vi "main_feedback_sliders.vi"(9 "Running?":refnum<vi>, 10 "Inflow fractions":refnum<vi>, 11 "PH":refnum<vi>) -> ()   [LabVIEW 2019]
uses:
  lib/libSimulationControl/libSimulationControl.lvlib
  lib/libFileFunctions/libFileFunctions.lvlib
panel:
  out "ph_arr out":dbl[](array[numeric])
  out "reactorState files":string
  out "Fractions":dbl[](array[numeric])
  out "Values":i32[](array[numeric])
  out "Sum":i32
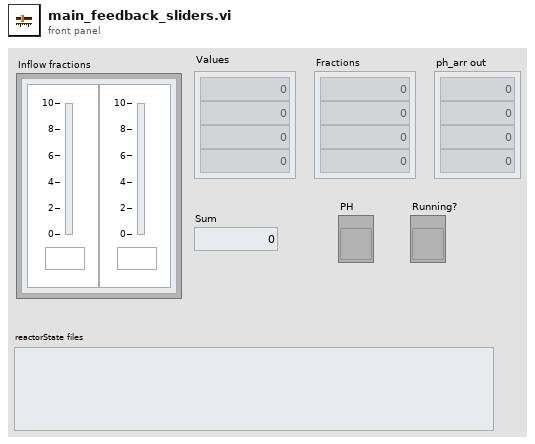
[diagram p1: front panel]
types:
  T1 = enum8{"Enabled", "Disabled", "Disabled and Grayed Out"}
  T2 = cluster{"Vertical Pointer Slide":i32, "String":string}
  T3 = cluster{"Vertical Pointer Slide":i32, "String":string}[]
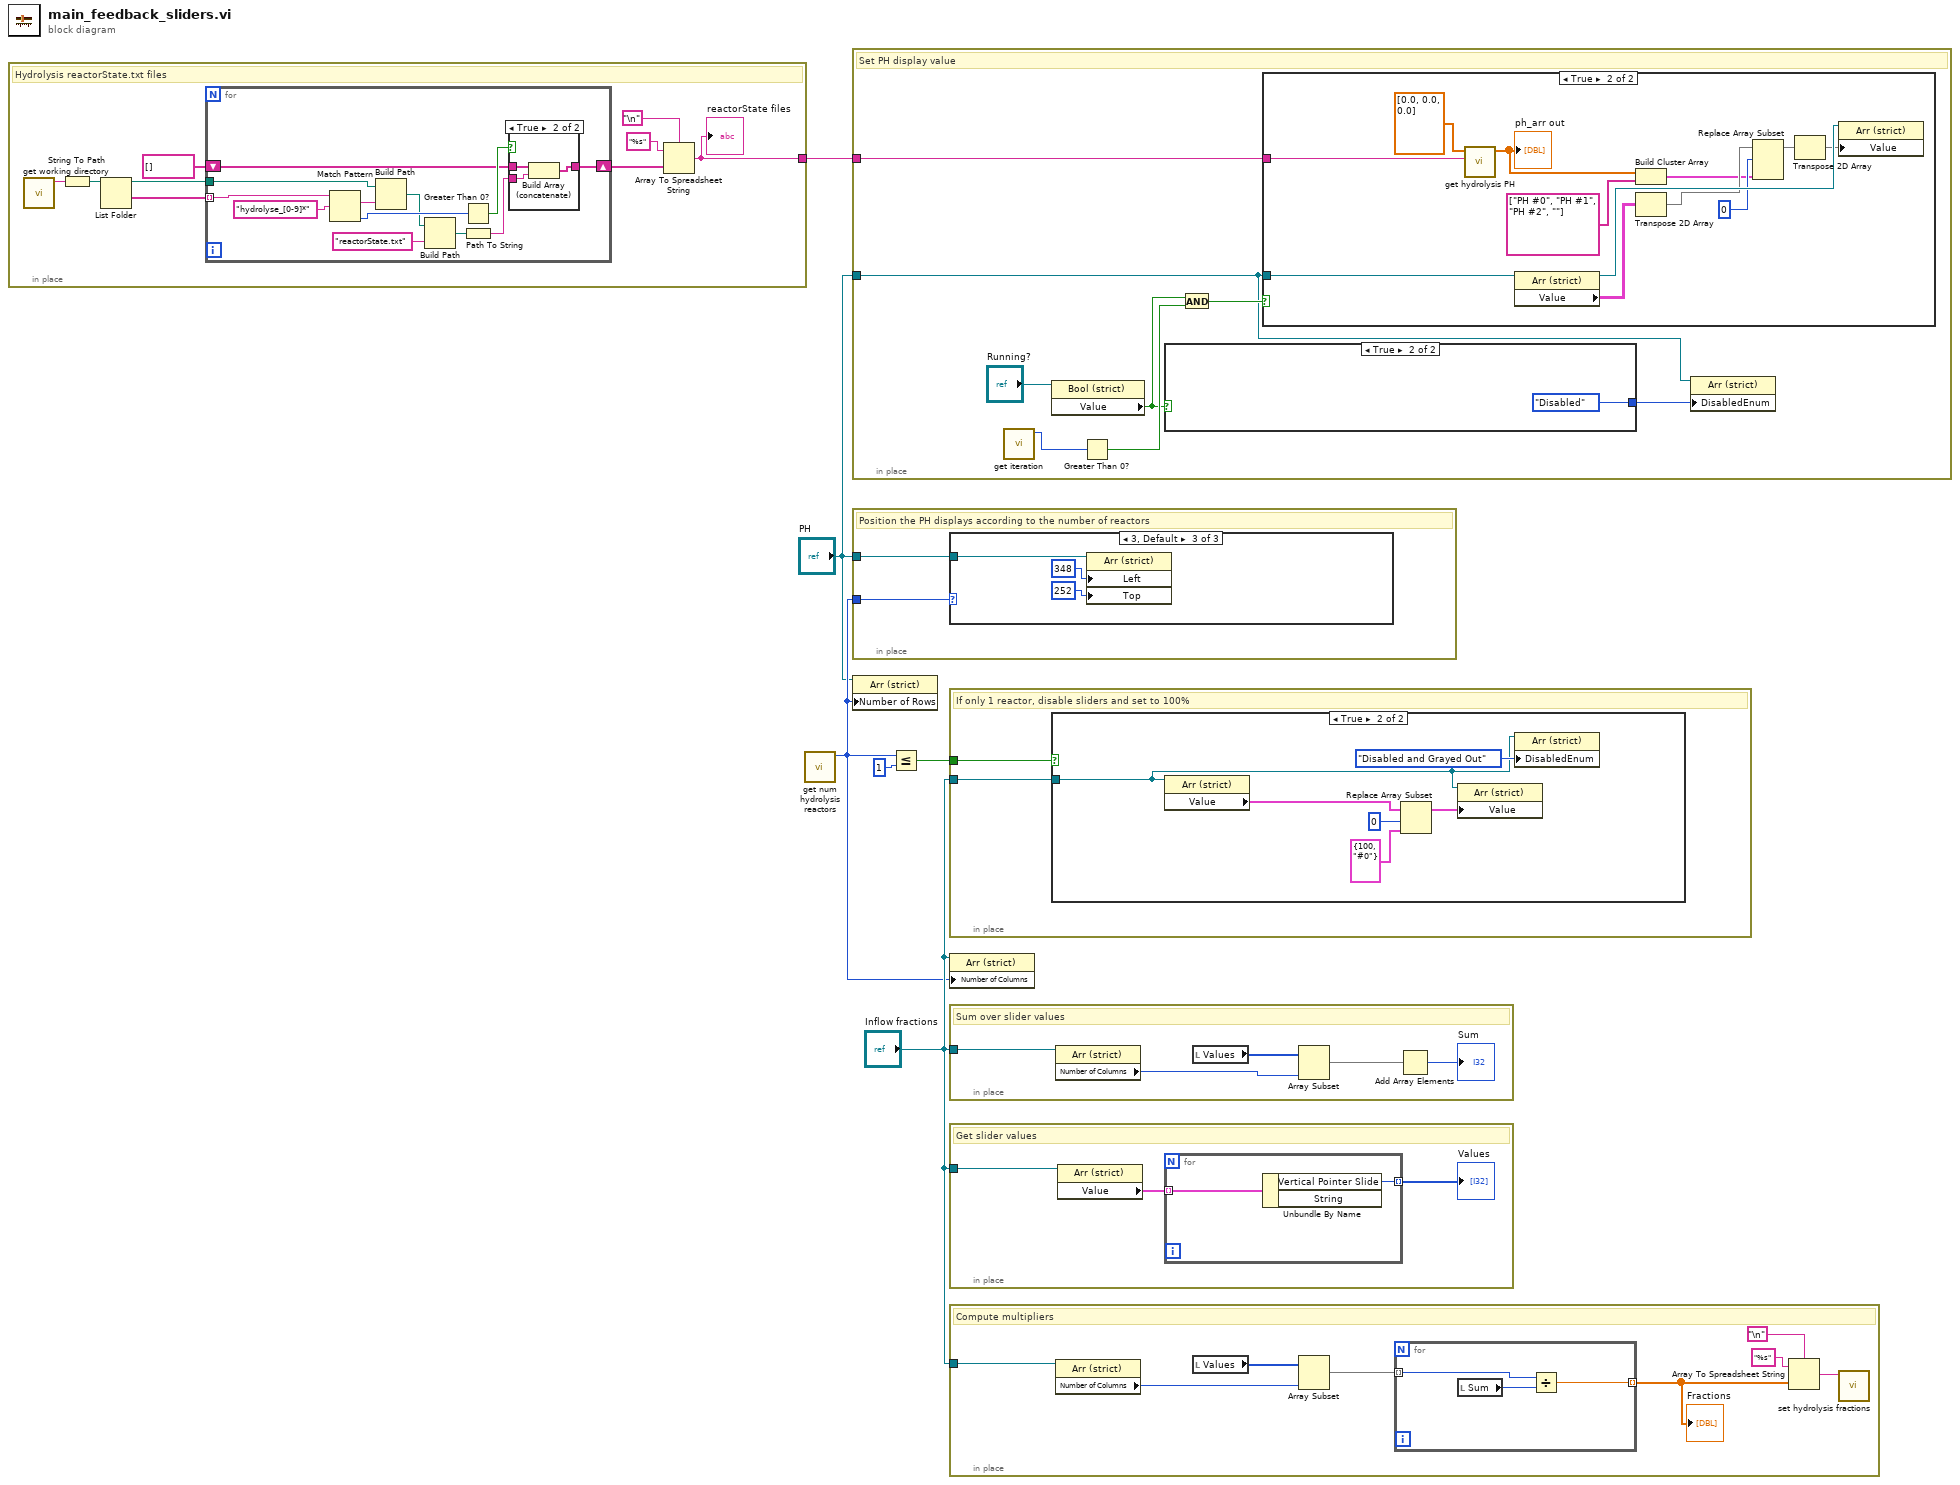
[diagram p0: block diagram]
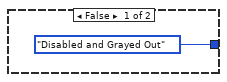
[diagram p3: hidden frame]
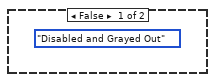
[diagram p4: hidden frame]
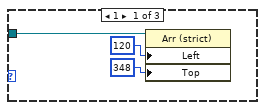
[diagram p5: hidden frame]
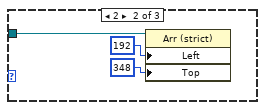
[diagram p6: hidden frame]
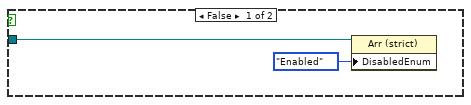
[diagram p7: hidden frame]
diagram:
  n1 = in-place {
    in-place-border: [w7] -> w1
    # "Hydrolysis reactorState.txt files"
    n2 = call "get working directory.vi"() -> ("function return"=w13:string)  [unwired: 10 in, 1 out]
    n3 = String To Path(string=w13) -> (path=w12:path)
    n4 = List Folder(path=w12) -> (path out=w11:path, folder names=w15:string[])  [unwired: 3 in, 2 out]
    n5 = for {
      tunnel: w15 -> [w22] mode=indexing
      shift-right: [w23] -> w10
      shift-left: string[] [] -> [w24]
      tunnel: w11 -> [w21]
      n6 = Match Pattern(string=w22, regular expression="hydrolyse_[0-9]*") -> (match substring=w20:string, offset past match=w25:i32)  [unwired: 1 in, 2 out]
      n7 = Build Path(base path=w21, name or relative path=w20) -> (appended path=w19:path)
      n8 = Build Path(base path=w19, name or relative path="reactorState.txt") -> (appended path=w17:path)
      n9 = Greater Than 0?(x=w25) -> (x > 0?=w26:bool)
      n10 = Path To String(path=w17) -> (string=w16:string)
      n11 = case shown="True" w26 {
        tunnel: [w28 w31] -> w23
        tunnel: w24 -> [w28 w30]
        tunnel: w16 -> [_ w29]
        frame False {
        }
        frame True {
          n12 = Build Array (concatenate)(w30, w29) -> (w31:string[])
        }
      }
    }
    n13 = Array To Spreadsheet String(delimiter (Tab)="\n", array=w10, 3:"%s" ("format string")) -> (spreadsheet string=w7:string)
    "reactorState files" <- w7
  }
  n14 = call "get num hydrolysis reactors.vi"() -> ("function return"=w3:i32)  [unwired: 10 in, 1 out]
  n15 = in-place {
    in-place-border: "PH" -> [w32]
    in-place-border: w1 -> [w36]
    # "Set PH display value"
    n16 = call "get iteration.vi"() -> ("function return"=w39:i32)  [unwired: 10 in, 1 out]
    n17 = property on="Property Node" class="Bool (strict)"(reference="Running?") -> ("Value"=w35:bool)  [unwired: 1 in, 2 out]
    n18 = Greater Than 0?(x=w39) -> (x > 0?=w38:bool)
    n19 = case shown="True" w35 {
      tunnel: [T1."Disabled and Grayed Out" ("Disabled") T1."Disabled" ("Disabled")] -> w34
      frame False {
      }
      frame True {
      }
    }
    n20 = And(x=w35, y=w38) -> (x .and. y?=w37:bool)
    n21 = case shown="True" w37 {
      tunnel: w32 -> [_ w53]
      tunnel: w36 -> [_ w43]
      frame False {
        (unwired) T1."Disabled and Grayed Out" ("Disabled")
      }
      frame True {
        n22 = call "get hydrolysis PH.vi"("reactor_state_files"=w43, "ph_arr 2"=dbl[] [0.0, 0.0, 0.0]) -> ("ph_arr out"=w44:dbl[])  [unwired: 8 in, 1 out]
        "ph_arr out" <- w44
        n23 = property on="Property Node" class="Arr (strict)"(reference=w53) -> (reference out=w51:refnum<vi>, "Value"=w52:cluster{"Meter":dbl, "String":string}[][])  [unwired: 1 in, 1 out]
        n24 = Build Cluster Array(w44, string[] ["PH #0", "PH #1", "PH #2", ""] ("Set Names")) -> (w47:cluster{"Numeric":dbl, "String":string}[])
        n25 = Transpose 2D Array(2D array=w52) -> (transposed array=w50:cluster{"Meter":dbl, "String":string}[][])
        n26 = Replace Array Subset(array=w50, new element=w47, index (row)=0) -> (w46:cluster{"Meter":dbl, "String":string}[][])  [unwired: 1 in]
        n27 = Transpose 2D Array(2D array=w46) -> (transposed array=w45:cluster{"Meter":dbl, "String":string}[][])
        n28 = property on="Property Node" class="Arr (strict)"(reference=w51, "Value"=w45) -> ()  [unwired: 1 in, 2 out]
      }
    }
    n29 = property on="Property Node" class="Arr (strict)"(reference=w32, "DisabledEnum"=w34) -> ()  [unwired: 1 in, 2 out]
  }
  n30 = in-place {
    in-place-border: w3 -> [w55]
    in-place-border: "PH" -> [w54]
    # "Position the PH displays according to the number of reactors"
    n31 = case shown="3, Default" w55 {
      tunnel: w54 -> [w58 w61 w64]
      frame 1 {
        n32 = property class="Arr (strict)"(reference=w58, "Left"=120 ("Position:Left"), "Top"=348 ("Position:Top")) -> ()  [unwired: 1 in, 2 out]
      }
      frame 2 {
        n33 = property class="Arr (strict)"(reference=w61, "Left"=192 ("Position:Left"), "Top"=348 ("Position:Top")) -> ()  [unwired: 1 in, 2 out]
      }
      frame 3, Default {
        n34 = property class="Arr (strict)"(reference=w64, "Left"=348 ("Position:Left"), "Top"=252 ("Position:Top")) -> ()  [unwired: 1 in, 2 out]
      }
    }
  }
  n35 = property class="Arr (strict)"(reference="PH", "Number of Rows"=w3) -> ()  [unwired: 1 in, 2 out]
  n36 = Less Or Equal?(x=w3, y=u32 1) -> (x <= y?=w5:bool)
  n37 = in-place {
    in-place-border: w5 -> [w66]
    in-place-border: "Inflow fractions" -> [w65]
    # "If only 1 reactor, disable sliders and set to 100%"
    n38 = case shown="True" w66 {
      tunnel: w65 -> [w67 w73]
      frame False {
        n39 = property on="Property Node" class="Arr (strict)"(reference=w67, "DisabledEnum"=T1."Enabled" ("Disabled")) -> ()  [unwired: 1 in, 2 out]
      }
      frame True {
        n40 = property on="Property Node" class="Arr (strict)"(reference=w73) -> ("Value"=w70:T3)  [unwired: 1 in, 2 out]
        n41 = Replace Array Subset(array=w70, new element=T2 {"Vertical Pointer Slide"=100, "String"="#0"} ("new element/subarray"), index=0) -> (w69:T3)
        n42 = property on="Property Node" class="Arr (strict)"(reference=w73, "Value"=w69) -> ()  [unwired: 1 in, 2 out]
        n43 = property on="Property Node" class="Arr (strict)"(reference=w73, "DisabledEnum"=T1."Disabled and Grayed Out" ("Disabled")) -> ()  [unwired: 1 in, 2 out]
      }
    }
  }
  n44 = property on="Property Node" class="Arr (strict)"(reference="Inflow fractions", "Number of Columns"=w3) -> ()  [unwired: 1 in, 2 out]
  n45 = in-place {
    in-place-border: "Inflow fractions" -> [w77]
    # "Sum over slider values"
    n46 = property on="Property Node" class="Arr (strict)"(reference=w77) -> ("Number of Columns"=w79:u32)  [unwired: 1 in, 2 out]
    n47 = local read "Values"() -> (w76:i32[])
    n48 = Array Subset(array=w76, length=w79) -> (w75:i32[])  [unwired: 1 in]
    n49 = Add Array Elements(numeric array=w75) -> (sum=→"Sum":i32)
  }
  n50 = in-place {
    in-place-border: "Inflow fractions" -> [w81]
    # "Get slider values"
    n51 = property on="Property Node" class="Arr (strict)"(reference=w81) -> ("Value"=w80:T3)  [unwired: 1 in, 2 out]
    n52 = for {
      tunnel: w80 -> [w84] mode=indexing
      tunnel: [w83] -> w82 mode=indexing
      n53 = Unbundle By Name(w84) -> ("Vertical Pointer Slide"=w83:i32)  [unwired: 1 out]
    }
    "Values" <- w82
  }
  n54 = in-place {
    in-place-border: "Inflow fractions" -> [w89]
    # "Compute multipliers"
    n55 = property on="Property Node" class="Arr (strict)"(reference=w89) -> ("Number of Columns"=w90:u32)  [unwired: 1 in, 2 out]
    n56 = local read "Values"() -> (w92:i32[])
    n57 = Array Subset(array=w92, length=w90) -> (w91:i32[])  [unwired: 1 in]
    n58 = for {
      tunnel: w91 -> [w94] mode=indexing
      tunnel: [w93] -> w88 mode=indexing
      n59 = local read "Sum"() -> (w95:i32)
      n60 = Divide(x=w94, y=w95) -> (x/y=w93:dbl)
    }
    "Fractions" <- w88
    n61 = Array To Spreadsheet String(delimiter (Tab)="\n", array=w88, 3:"%s" ("format string")) -> (spreadsheet string=w87:string)
    n62 = call "set hydrolysis fractions.vi"("fract"=w87) -> ()  [unwired: 10 in, 1 out]
  }
